vi "Property Nodes graph.vi"() -> ()   [LabVIEW 2015]
panel:
  in  "Channel 3":bool
  in  "Channel 2":bool
  in  "Channel 1":bool
  in  "Clear":bool
  in  "stop":bool
  out "Waveform Chart":cluster{dbl, dbl, dbl}(graph)
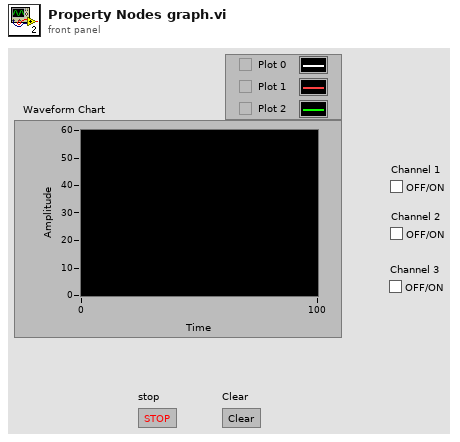
[diagram p1: front panel]
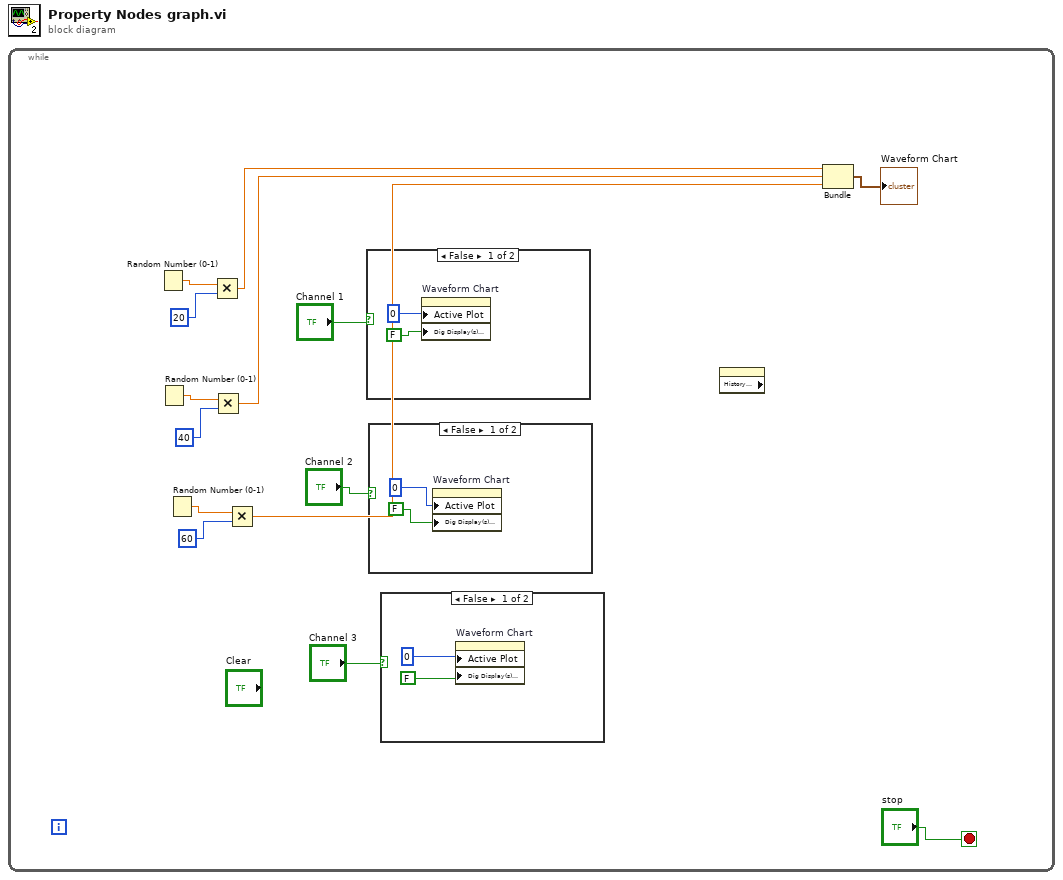
[diagram p0: block diagram]
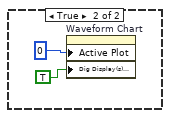
[diagram p2: hidden frame]
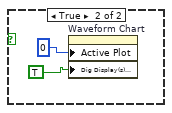
[diagram p3: hidden frame]
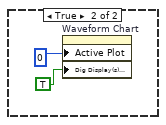
[diagram p4: hidden frame]
diagram:
  n1 = while {
    stop <- "stop" stop-if-true
    n2 = Random Number (0-1) ("Random Number (0-40)")() -> (number: 0 to 1=w13:dbl)
    n3 = Random Number (0-1) ("Random Number (0-20)")() -> (number: 0 to 1=w8:dbl)
    n4 = Random Number (0-1) ("Random Number (0-100)")() -> (number: 0 to 1=w5:dbl)
    n5 = Multiply(x=w13, y=20) -> (x*y=w10:dbl)
    n6 = Multiply(x=w8, y=40) -> (x*y=w7:dbl)
    n7 = Multiply(x=w5, y=60) -> (x*y=w4:dbl)
    n8 = case shown="False" "Channel 1" {
      frame False {
        n9 = property on="Waveform Chart" class="WFChart (strict)"("Active Plot"=0, "Dig Display(s) Visible"=FALSE) -> ()  [unwired: 2 in, 2 out]
      }
      frame True {
        n10 = property on="Waveform Chart" class="WFChart (strict)"("Active Plot"=0, "Dig Display(s) Visible"=TRUE) -> ()  [unwired: 2 in, 2 out]
      }
    }
    n11 = case shown="False" "Channel 2" {
      frame False {
        n12 = property on="Waveform Chart" class="WFChart (strict)"("Active Plot"=0, "Dig Display(s) Visible"=FALSE) -> ()  [unwired: 2 in, 2 out]
      }
      frame True {
        n13 = property on="Waveform Chart" class="WFChart (strict)"("Active Plot"=0, "Dig Display(s) Visible"=TRUE) -> ()  [unwired: 2 in, 2 out]
      }
    }
    n14 = case shown="False" "Channel 3" {
      frame False {
        n15 = property on="Waveform Chart" class="WFChart (strict)"("Active Plot"=0, "Dig Display(s) Visible"=FALSE) -> ()  [unwired: 2 in, 2 out]
      }
      frame True {
        n16 = property on="Waveform Chart" class="WFChart (strict)"("Active Plot"=0, "Dig Display(s) Visible"=TRUE) -> ()  [unwired: 2 in, 2 out]
      }
    }
    n17 = property class="WFChart (strict)" props=["History Data"]() -> ()  [unwired: 2 in, 3 out]
    n18 = Bundle(w10, w7, w4) -> (→"Waveform Chart":cluster{dbl, dbl, dbl})  [unwired: 1 in]
  }
